vi "FPGAcode_check_velocity.vi"() -> ()   [LabVIEW 2015]
uses:
  <vilib>/Platform/TimedLoop/XDataNode/timing_clust.ctl
  <vilib>/Platform/TimedLoop/XDataNode/nitl_modes.ctl
  <vilib>/Platform/TimedLoop/XDataNode/wakeup.ctl
  <vilib>/rvi/eio/common/nirviEmuTemplateMethod_errors.vi
  <vilib>/rvi/Emulation/niFpgaGetClockAttributes.vi
  <vilib>/rvi/Emulation/niFpgaSctlEmulationGetInTimedLoop.vi
  <vilib>/rvi/Emulation/niFpgaEmulationReportErrorSimple.vi
  <vilib>/rvi/Emulation/niFpgaProcessEmulError.vi
  <vilib>/rvi/Emulation/niFpgaCriticalErrorInLSC.vi
  <vilib>/eio/EIONode/EIONode.xnode
  <vilib>/Platform/TimedLoop/XDataNode/XDataNode.xnode
  <vilib>/Platform/TimedLoop/XDataNode/XDNodeRunTimeDep.lvlib
panel:
  out "Check Data?":bool
  out "Filter":i16
  out "Vel Count 7":i32
  out "Vel Count 6":i32
  out "Vel Count 5":i32
  out "Vel Count 4":i32
  out "Vel Count 3":i32
  out "Vel Count 2":i32
  out "Vel Count 1":i32
  out "Filter 1 Detector 3 Correlation":i32
  in  "Filter 2 threshold":i32=1000
  out "Filter 2 Detector 3 Correlation":i32
  in  "Filter 1 threshold":i32=1000
  in  "Filter 3 threshold":i32=1000
  out "Filter 3 Detector 3 Correlation":i32
  in  "Filter 4 threshold":i32=1000
  out "Filter 4 Detector 3 Correlation":i32
  in  "Filter 5 threshold":i32
  out "Filter 5 Detector 3 Correlation":i32
  in  "Filter 6 threshold":i32
  out "Filter 6 Detector 3 Correlation":i32
  in  "Filter 7 threshold":i32
  out "Filter 7 Detector 3 Correlation":i32
  out "Plates":bool
  in  "High Charge Limit":i16
  in  "Low Charge Limit":i16
  in  "High Velocity Count":i32
  in  "Low Velocity Count":i32
  in  "High Mass Limit":i64
  in  "Low Mass Limit":i64
  in  "Mult1":fxp<+,16,7>
  out "Delay1":bool
  in  "One Shot":bool
  out "Not Armed?":bool
  in  "Reset One Shot":bool
  out "Del Not Armed?":bool
  out "IO Module\\AI 0":i16
  out "IO Module\\AI 1":i16
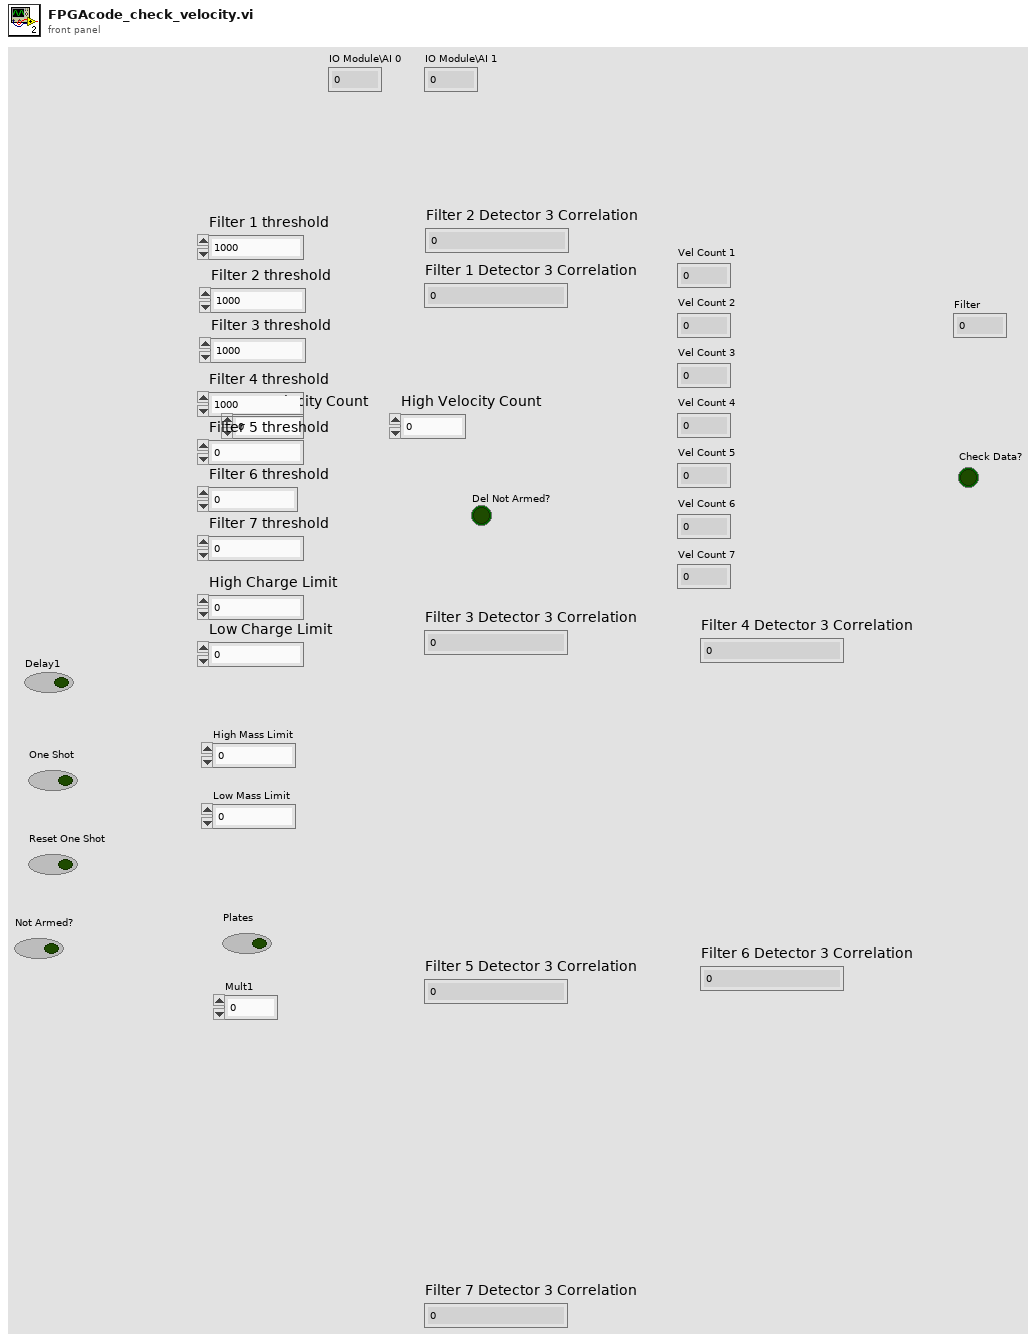
[diagram p1: front panel]
types:
  T1 = typedef "XDNodeRunTimeDep.lvlib/timing_clust.ctl" = cluster{"Expected End [f-1]":u64, "Actual End [f-1]":u64, "Finished Late? [f-1]":bool, "Expected End [i-1]":u64, "Actual End [i-1]":u64, "Finished Late? [i-1]":bool, "Expected Start [i]":u64, "Actual Start [i]":u64, "Expected Start [f]":u64, "Actual Start [f]":u64, "Source Name":string, "Structure Name":string, "Period":i64, "Deadline":i64, "Offset":i64, "Start":i64, "Priority":i32, "Timeout":i32, "Mode":T2, "Wakeup Reason":T3, "Error":errorcluster, "Source Type":string, "Secondary Source Type":string, "Global End Time":u64, "Global Start Time":u64, "Frame Duration":u64, "Iteration Duration":u64, "Assigned CPU":i32, "I/O Scan Engine Mode":u32}
  T2 = typedef "XDNodeRunTimeDep.lvlib/nitl_modes.ctl" = enum32{"No Change", "Process missed periods, maintain original phase", "Discard missed periods, maintain original phase", "Process missed periods, ignore original phase", "Discard missed periods, ignore original phase"}
  T3 = typedef "XDNodeRunTimeDep.lvlib/wakeup.ctl" = enum32{"Normal", "Aborted", "Asynchronous wakeup", "Timing source error", "Timed loop error", "Timeout"}
  T4 = cluster{"Separation cut off 1":i32, "Filter Number":i32, "Separation cut off 2":i32}
  T5 = cluster{"Old Average":i32, "New Average":i32, "Current State":u8, "Detector 1 Correlation":i32, "Detector 3 Correlation":i32, "Velocity Count":i32, "Detector Counter in":i32, "Timeout Count in":i32, "Measured Charge in":i32, "Filter Threshold":i32, "High Correlation in":i32, "Offset":i32, "Offset Average":i32, "Measured Velocity In":i32, "Mult Cluster":cluster{"Mult1":fxp<+,16,7>, "Mult1 Use?":bool}, "Final Delay Count In":u16, "Delay1 In":i32}
  T6 = cluster{"High Charge Limit":i16, "Low Charge Limit":i16, "Low Velocity Count":i32, "High Velocity Count":i32, "Low Velocity Count":i32, fxp<+,30,25>, "High Mass Limit":i64, "Low Mass Limit":i64}
  T7 = cluster{"Average Out":i32, "Next State":u8, "Velocity Count out":i32, "Detector counter out":i32, "Timeout count out":u32, "Measured Charge Out":i32, "High Correlation Out":i32, "Plates":bool, "Offset Out":i32, "Measured Velocity Out":i32, "Final Delay Count Out":u16, "Out1":bool, "Delay1":i32}
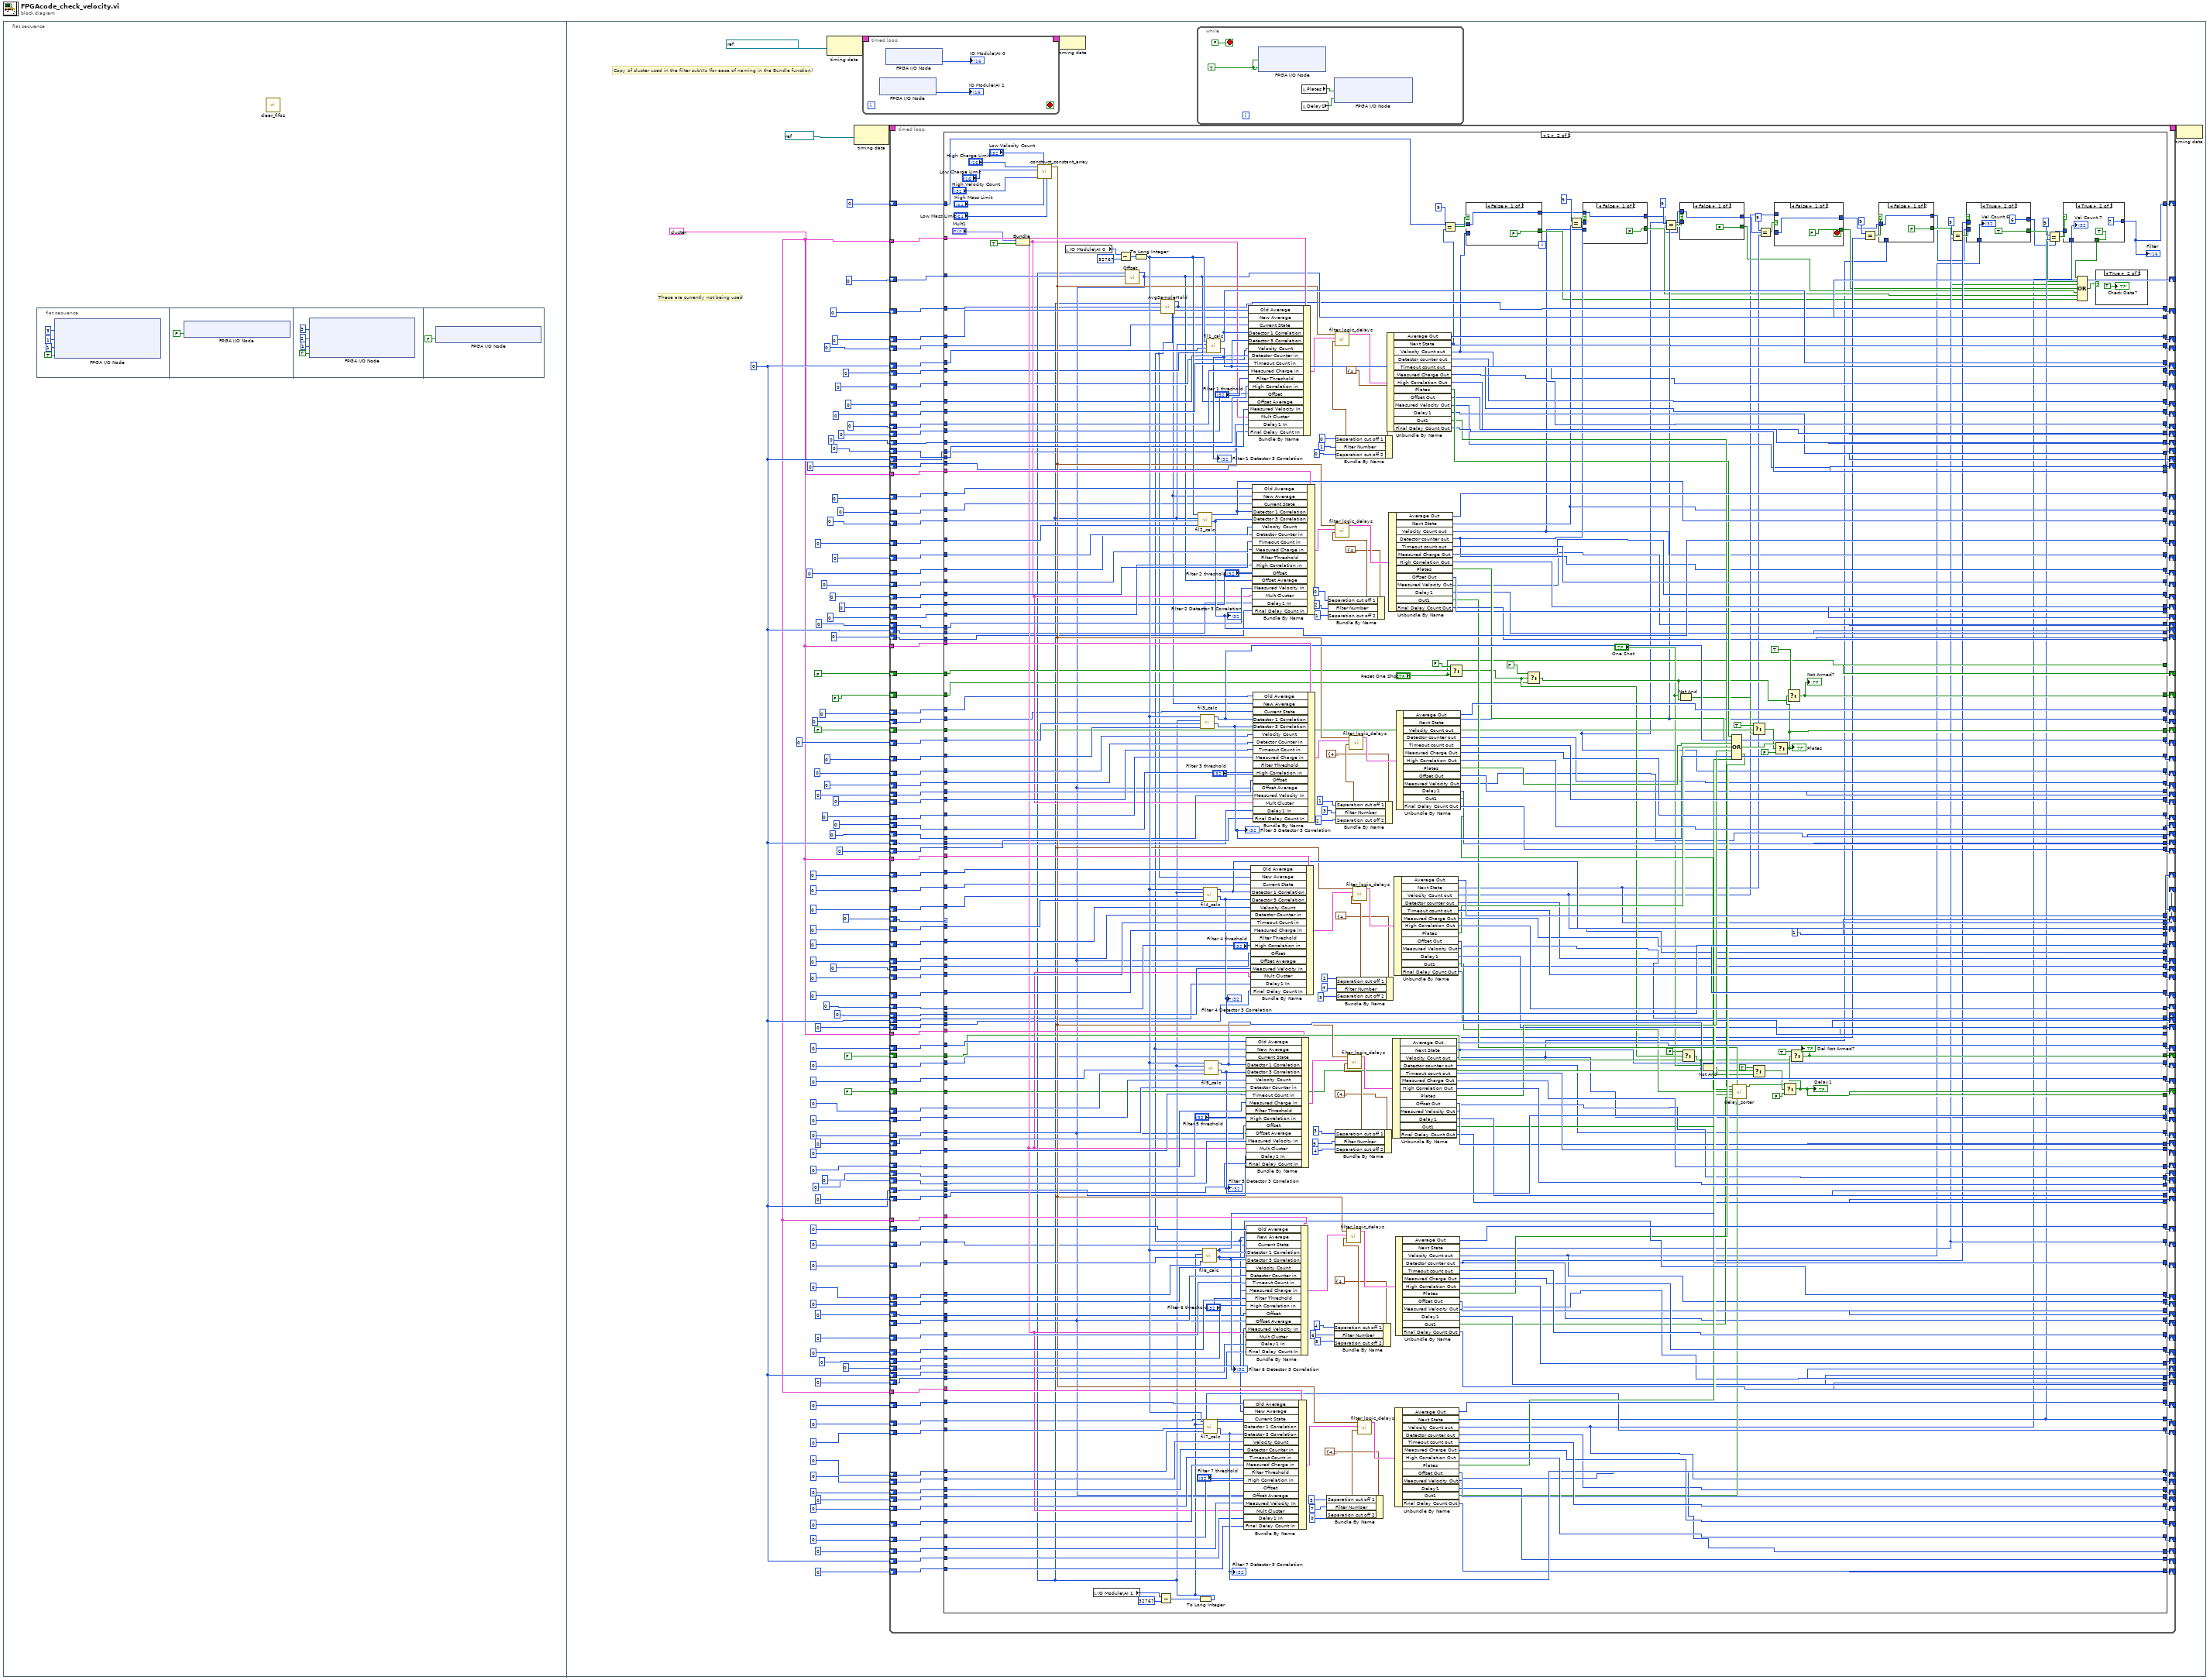
[diagram p0: block diagram]
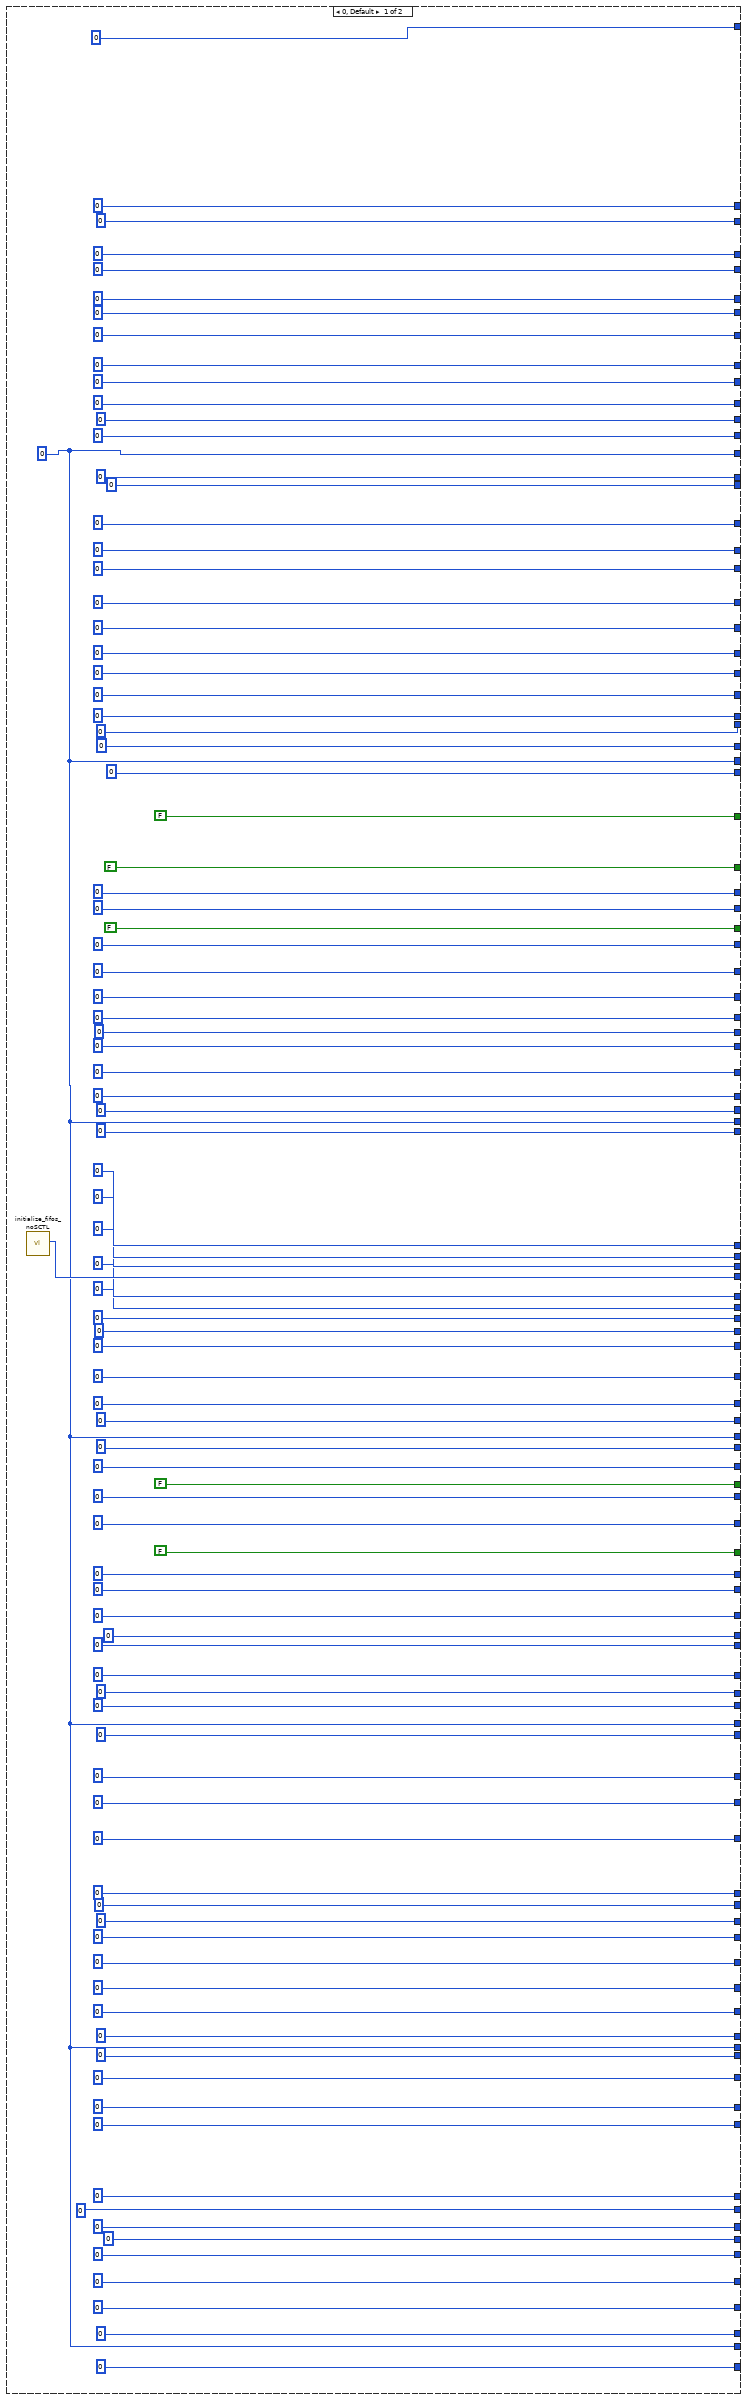
[diagram p2: hidden frame]
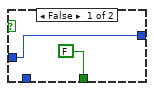
[diagram p4: hidden frame]
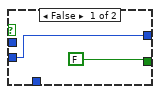
[diagram p5: hidden frame]
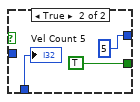
[diagram p6: hidden frame]
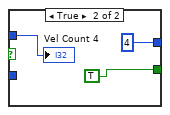
[diagram p7: hidden frame]
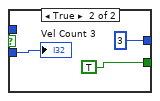
[diagram p8: hidden frame]
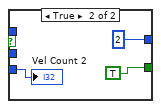
[diagram p9: hidden frame]
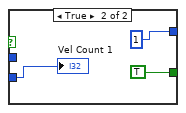
[diagram p10: hidden frame]
diagram:
  n1 = flat-sequence {
    frame #0 {
      n2 = flat-sequence {
        frame #0 {
          n3 = xnode "FPGA I/O Node"("IO Module\\User Command"=u8 3 ("IO Module\\User Command"), "IO Module\\User Data 0"=u8 1 ("IO Module\\User Data 0"), "IO Module\\User Data 1"=u8 1 ("IO Module\\User Data 1"), "IO Module\\User Command Commit"=TRUE ("IO Module\\User Command Commit")) -> ()  [unwired: 4 in, 4 out]
        }
        frame #1 {
          n4 = xnode "FPGA I/O Node"("IO Module\\User Command Commit"=FALSE ("IO Module\\User Command Commit")) -> ()  [unwired: 1 in, 1 out]
        }
        frame #2 {
          n5 = xnode "FPGA I/O Node"("IO Module\\User Command"=u8 3 ("IO Module\\User Command"), "IO Module\\User Data 0"=u8 2 ("IO Module\\User Data 0"), "IO Module\\User Data 1"=u8 1 ("IO Module\\User Data 1"), "IO Module\\User Command Commit"=TRUE ("IO Module\\User Command Commit")) -> ()  [unwired: 4 in, 4 out]
        }
        frame #3 {
          n6 = xnode "FPGA I/O Node"("IO Module\\User Command Commit"=FALSE ("IO Module\\User Command Commit")) -> ()  [unwired: 1 in, 1 out]
        }
      }
      n7 = call "clear_fifos.vi"() -> ()  [unwired: 1 in]
    }
    frame #1 {
      w16 = T5 {"Old Average"=0, "New Average"=0, "Current State"=0, "Detector 1 Correlation"=0, "Detector 3 Correlation"=0, "Velocity Count"=0, "Detector Counter in"=0, "Timeout Count in"=0, "Measured Charge in"=0, "Filter Threshold"=0, "High Correlation in"=0, "Offset"=0, "Offset Average"=0, "Measured Velocity In"=0, "Mult Cluster"={"Mult1"=0.0, "Mult1 Use?"=FALSE}, "Final Delay Count In"=0, "Delay1 In"=0} ("Variables Cluster")
      w19 = 0 ("Detector 1 Correlation Out")
      # "These are currently not being used"
      # "Copy of cluster used in the filter subVIs (for ease of naming in the Bundle function)"
      n8 = node-c288(refnum<k21> "IO Module\\Sample Clock" ("Source Name")) -> (w45:T1)
      n9 = node-c288(refnum<k21> "26MHz" ("Source Name")) -> (w109:T1)
      n10 = timed-loop {
        timing: w45 -> [_]
        timing-out: [_] -> w44
        stop <- _ stop-if-true
        n11 = xnode "FPGA I/O Node"() -> ("IO Module\\AI 2"=→"IO Module\\AI 1":u16)  [unwired: 1 in, 1 out]
        n12 = xnode "FPGA I/O Node"() -> ("IO Module\\AI 1"=→"IO Module\\AI 0":u16)  [unwired: 1 in, 1 out]
      }
      n13 = timed-loop {
        timing: w109 -> [_]
        timing-out: [_] -> w108
        shift-right: [w321] -> _
        shift-left: 0 ("Velocity Count out") -> [w243]
        shift-right: [w322] -> _
        shift-left: 0 ("Detector 1 Correlation out") -> [w244]
        shift-right: [w208] -> _
        shift-left: 0 ("Detector counter out") -> [w245]
        shift-right: [w239] -> _
        shift-left: 0 ("Next State") -> [w246]
        shift-right: [w207] -> _
        shift-left: 0 ("Detector 3 Correlation out") -> [w242]
        shift-right: [w320] -> _
        shift-left: 0 ("Timeout count out") -> [w241]
        shift-right: [w235] -> _
        shift-left: 0 ("Next State") -> [w238]
        shift-right: [w234] -> _
        shift-left: 0 ("Detector counter out") -> [w237]
        shift-right: [w206] -> _
        shift-left: 0 ("Detector 1 Correlation out") -> [w314]
        shift-right: [w311] -> _
        shift-left: 0 ("Velocity Count out") -> [w313]
        shift-right: [w310] -> _
        shift-left: u32 0 ("Detector 3 Correlation out") -> [w312]
        shift-right: [w305] -> _
        shift-left: 0 ("Timeout count out") -> [w306]
        shift-right: [w229] -> _
        shift-left: 0 ("Next State") -> [w232]
        shift-right: [w204] -> _
        shift-left: 0 ("Detector counter out") -> [w302]
        shift-right: [w300] -> _
        shift-left: 0 ("Detector 1 Correlation out") -> [w301]
        shift-right: [w298] -> _
        shift-left: u32 0 ("Velocity Count out") -> [w299]
        shift-right: [w203] -> _
        shift-left: 0 ("Detector 3 Correlation out") -> [w297]
        shift-right: [w296] -> _
        shift-left: 0 ("Timeout count out") -> [w231]
        shift-right: [w323] -> _
        shift-left: u8 0 ("High Correlation Out") -> [w326]
        shift-right: [w315] -> _
        shift-left: u8 0 ("High Correlation Out") -> [w316]
        shift-right: [w230] -> _
        shift-left: 0 ("High Correlation Out") -> [w233]
        shift-right: [w324] -> _
        shift-left: 0 ("Measured Charge Out") -> [w327]
        shift-right: [w317] -> _
        shift-left: 0 ("Measured Charge Out") -> [w318]
        shift-right: [w304] -> _
        shift-left: u8 0 ("Measured Charge Out") -> [w303]
        shift-right: [w194] -> _
        shift-left: 0 ("Output New Average") -> [w328]
        shift-right: [w240] -> _
        shift-left: w19 -> [w247]
        tunnel: w16 -> [w325]
        shift-right: [w205] -> _
        shift-left: 0 ("High Sample Out") -> [w308]
        shift-right: [w309] -> _
        shift-left: 0 ("High Correlation Out") -> [w236]
        tunnel: w16 -> [w319]
        tunnel: w16 -> [w307]
        shift-right: [w295] -> _
        shift-left: 0 ("Average Out") -> [w294]
        shift-right: [w293] -> _
        shift-left: u8 0 ("Next State") -> [w292]
        shift-right: [w225] -> _
        shift-left: 0 ("Detector 1 Correlation out") -> [w227]
        shift-right: [w224] -> _
        shift-left: 0 ("Detector 3 Correlation out") -> [w226]
        shift-right: [w202] -> _
        shift-left: 0 ("Velocity Count out") -> [w291]
        shift-right: [w290] -> _
        shift-left: 0 ("Detector counter out") -> [w289]
        shift-right: [w288] -> _
        shift-left: u32 0 ("Timeout count out") -> [w287]
        shift-right: [w201] -> _
        shift-left: 0 ("Measured Charge Out") -> [w286]
        shift-right: [w285] -> _
        shift-left: 0 ("High Correlation Out") -> [w228]
        tunnel: w16 -> [w284]
        shift-right: [w282] -> _
        shift-left: 0 ("Average Out") -> [w281]
        shift-right: [w280] -> _
        shift-left: u8 0 ("Next State") -> [w279]
        shift-right: [w220] -> _
        shift-left: 0 ("Detector 1 Correlation out") -> [w223]
        shift-right: [w219] -> _
        shift-left: 0 ("Detector 3 Correlation out") -> [w222]
        shift-right: [w200] -> _
        shift-left: 0 ("Velocity Count out") -> [w278]
        shift-right: [w277] -> _
        shift-left: 0 ("Detector counter out") -> [w276]
        shift-right: [w275] -> _
        shift-left: u32 0 ("Timeout count out") -> [w274]
        shift-right: [w199] -> _
        shift-left: 0 ("Measured Charge Out") -> [w273]
        shift-right: [w272] -> _
        shift-left: 0 ("High Correlation Out") -> [w221]
        tunnel: w16 -> [w283]
        shift-right: [w270] -> _
        shift-left: 0 ("Average Out") -> [w268]
        shift-right: [w269] -> _
        shift-left: u8 0 ("Next State") -> [w265]
        shift-right: [w215] -> _
        shift-left: 0 ("Detector 1 Correlation out") -> [w218]
        shift-right: [w214] -> _
        shift-left: 0 ("Detector 3 Correlation out") -> [w217]
        shift-right: [w197] -> _
        shift-left: 0 ("Velocity Count out") -> [w267]
        shift-right: [w264] -> _
        shift-left: _ -> [w266]
        shift-right: [w263] -> _
        shift-left: u32 0 ("Timeout count out") -> [w262]
        shift-right: [w198] -> _
        shift-left: 0 ("Measured Charge Out") -> [w261]
        shift-right: [w260] -> _
        shift-left: 0 ("High Correlation Out") -> [w216]
        tunnel: w16 -> [w271]
        shift-right: [w258] -> _
        shift-left: 0 ("Average Out") -> [w257]
        shift-right: [w256] -> _
        shift-left: u8 0 ("Next State") -> [w248]
        shift-right: [w210] -> _
        shift-left: 0 ("Detector 1 Correlation out") -> [w213]
        shift-right: [w209] -> _
        shift-left: 0 ("Detector 3 Correlation out") -> [w212]
        shift-right: [w196] -> _
        shift-left: 0 ("Velocity Count out") -> [w255]
        shift-right: [w254] -> _
        shift-left: 0 ("Detector counter out") -> [w253]
        shift-right: [w252] -> _
        shift-left: u32 0 ("Timeout count out") -> [w251]
        shift-right: [w195] -> _
        shift-left: 0 ("Measured Charge Out") -> [w250]
        shift-right: [w249] -> _
        shift-left: 0 ("High Correlation Out") -> [w211]
        tunnel: w16 -> [w259]
        shift-right: [w192] -> _
        shift-left: i16 0 -> [w193]
        shift-right: [w190] -> _
        shift-left: 0 -> [w191]
        shift-right: [w189] -> _
        shift-left: 0 -> [w186]
        shift-right: [w187] -> _
        shift-left: 0 -> [w188]
        shift-right: [w184] -> _
        shift-left: 0 ("Offset Out") -> [w185]
        shift-right: [w183] -> _
        shift-left: 0 ("Offset Out") -> [w182]
        shift-right: [w181] -> _
        shift-left: 0 ("Offset Out") -> [w180]
        shift-right: [w179] -> _
        shift-left: 0 ("Offset Out") -> [w178]
        shift-right: [w177] -> _
        shift-left: 0 ("Offset Out") -> [w176]
        shift-right: [w174] -> _
        shift-left: 0 -> [w175]
        shift-right: [w173] -> _
        shift-left: 0 -> [w162]
        shift-right: [w172] -> _
        shift-left: 0 -> [w163]
        shift-right: [w171] -> _
        shift-left: 0 -> [w164]
        shift-right: [w170] -> _
        shift-left: 0 -> [w165]
        shift-right: [w169] -> _
        shift-left: 0 -> [w166]
        shift-right: [w168] -> _
        shift-left: 0 ("Measured Velocity Out") -> [w167]
        shift-right: [w161] -> _
        shift-left: w19 -> [w159]
        shift-right: [w160] -> _
        shift-left: u32 0 ("Final Delay Count Out") -> [w158]
        shift-right: [w157] -> _
        shift-left: w19 -> [w155]
        shift-right: [w156] -> _
        shift-left: u32 0 ("Final Delay Count Out") -> [w154]
        shift-right: [w153] -> _
        shift-left: w19 -> [w151]
        shift-right: [w152] -> _
        shift-left: u32 0 ("Final Delay Count Out") -> [w150]
        shift-right: [w149] -> _
        shift-left: w19 -> [w147]
        shift-right: [w148] -> _
        shift-left: u32 0 ("Final Delay Count Out") -> [w146]
        shift-right: [w145] -> _
        shift-left: w19 -> [w143]
        shift-right: [w144] -> _
        shift-left: u32 0 ("Final Delay Count Out") -> [w142]
        shift-right: [w141] -> _
        shift-left: w19 -> [w139]
        shift-right: [w140] -> _
        shift-left: u32 0 ("Final Delay Count Out") -> [w138]
        shift-right: [w137] -> _
        shift-left: w19 -> [w135]
        shift-right: [w136] -> _
        shift-left: u32 0 ("Final Delay Count Out") -> [w134]
        shift-right: [w132] -> _
        shift-left: FALSE -> [w133]
        shift-right: [w131] -> _
        shift-left: FALSE ("f") -> [w130]
        shift-right: [w129] -> _
        shift-left: FALSE ("Reset One Shot") -> [w128]
        shift-right: [w124] -> _
        shift-left: FALSE -> [w127]
        shift-right: [w125] -> _
        shift-left: FALSE -> [w126]
        shift-right: [w123] -> _
        shift-left: i16 0 ("Filter") -> [w122]
        stop <- _ stop-if-true
        n14 = case shown="1" w193 {
          tunnel: w328 -> [_ w491]
          tunnel: w327 -> [_ w763]
          tunnel: w326 -> [_ w458]
          tunnel: w325 -> [_ w762]
          tunnel: [0 ("Average Out") w761] -> w324
          tunnel: [u16 0 ("Next State") w488] -> w323
          tunnel: [0 ("Detector counter out") w481] -> w322
          tunnel: [u32 0 ("Timeout count out") w760] -> w321
          tunnel: [0 ("High Correlation Out") w759] -> w320
          tunnel: w319 -> [_ w758]
          tunnel: w318 -> [_ w757]
          tunnel: [0 ("Average Out") w756] -> w317
          tunnel: w316 -> [_ w457]
          tunnel: [u16 0 ("Next State") w480] -> w315
          tunnel: w314 -> [_ w755]
          tunnel: w313 -> [_ w617]
          tunnel: w312 -> [_ w754]
          tunnel: [0 ("Detector counter out") w479] -> w311
          tunnel: [u32 0 ("Timeout count out") w753] -> w310
          tunnel: [0 ("High Correlation Out") w752] -> w309
          tunnel: w308 -> [_ w751]
          tunnel: w307 -> [_ w750]
          tunnel: w306 -> [_ w749]
          tunnel: [0 ("Average Out") w748] -> w305
          tunnel: [u16 0 ("Next State") w477] -> w304
          tunnel: w303 -> [_ w456]
          tunnel: w302 -> [_ w747]
          tunnel: w301 -> [_ w616]
          tunnel: [0 ("Detector counter out") w476] -> w300
          tunnel: w299 -> [_ w746]
          tunnel: [u32 0 ("Timeout count out") w745] -> w298
          tunnel: w297 -> [_ w744]
          tunnel: [0 ("High Correlation Out") w743] -> w296
          tunnel: [0 ("Average Out") w742] -> w295
          tunnel: w294 -> [_ w741]
          tunnel: [u16 0 ("Next State") w466] -> w293
          tunnel: w292 -> [_ w455]
          tunnel: w291 -> [_ w740]
          tunnel: [0 ("Detector counter out") w465] -> w290
          tunnel: w289 -> [_ w615]
          tunnel: [u32 0 ("Timeout count out") w739] -> w288
          tunnel: w287 -> [_ w738]
          tunnel: w286 -> [_ w737]
          tunnel: [0 ("High Correlation Out") w736] -> w285
          tunnel: w284 -> [_ w735]
          tunnel: w283 -> [_ w734]
          tunnel: [0 ("Average Out") w733] -> w282
          tunnel: w281 -> [_ w732]
          tunnel: [u16 0 ("Next State") w464] -> w280
          tunnel: w279 -> [_ w454]
          tunnel: w278 -> [_ w731]
          tunnel: [0 ("Detector counter out") w463] -> w277
          tunnel: w276 -> [_ w614]
          tunnel: [u32 0 ("Timeout count out") w730] -> w275
          tunnel: w274 -> [_ w729]
          tunnel: w273 -> [_ w728]
          tunnel: [0 ("High Correlation Out") w727] -> w272
          tunnel: w271 -> [_ w726]
          tunnel: [0 ("Average Out") w725] -> w270
          tunnel: [u16 0 ("Next State") w462] -> w269
          tunnel: w268 -> [_ w724]
          tunnel: w267 -> [_ w723]
          tunnel: w266 -> [_ w613]
          tunnel: w265 -> [_ w453]
          tunnel: [0 ("Detector counter out") w461] -> w264
          tunnel: [u32 0 ("Timeout count out") w722] -> w263
          tunnel: w262 -> [_ w721]
          tunnel: w261 -> [_ w720]
          tunnel: [0 ("High Correlation Out") w719] -> w260
          tunnel: w259 -> [_ w718]
          tunnel: [0 ("Average Out") w717] -> w258
          tunnel: w257 -> [_ w716]
          tunnel: [u16 0 ("Next State") w460] -> w256
          tunnel: w255 -> [_ w715]
          tunnel: [0 ("Detector counter out") w459] -> w254
          tunnel: w253 -> [_ w612]
          tunnel: [u32 0 ("Timeout count out") w714] -> w252
          tunnel: w251 -> [_ w713]
          tunnel: w250 -> [_ w712]
          tunnel: [0 ("High Correlation Out") w711] -> w249
          tunnel: w248 -> [_ w452]
          tunnel: w247 -> [_ w710]
          tunnel: w246 -> [_ w530]
          tunnel: w245 -> [_ w531]
          tunnel: w244 -> [_ w618]
          tunnel: w243 -> [_ w709]
          tunnel: w242 -> [_ w708]
          tunnel: w241 -> [_ w707]
          tunnel: [0 ("Detector 1 Correlation Out") w706] -> w240
          tunnel: [0 ("Detector 3 Correlation Out") w705] -> w239
          tunnel: w238 -> [_ w704]
          tunnel: w237 -> [_ w703]
          tunnel: w236 -> [_ w702]
          tunnel: [0 ("Detector 1 Correlation Out") w701] -> w235
          tunnel: [0 ("Detector 3 Correlation Out") w700] -> w234
          tunnel: w233 -> [_ w699]
          tunnel: w232 -> [_ w698]
          tunnel: w231 -> [_ w697]
          tunnel: [0 ("Detector 1 Correlation Out") w696] -> w230
          tunnel: [0 ("Detector 3 Correlation Out") w695] -> w229
          tunnel: w228 -> [_ w694]
          tunnel: w227 -> [_ w693]
          tunnel: w226 -> [_ w692]
          tunnel: [0 ("Detector 1 Correlation Out") w691] -> w225
          tunnel: [0 ("Detector 3 Correlation Out") w690] -> w224
          tunnel: w223 -> [_ w689]
          tunnel: w222 -> [_ w688]
          tunnel: w221 -> [_ w687]
          tunnel: [0 ("Detector 1 Correlation Out") w686] -> w220
          tunnel: [0 ("Detector 3 Correlation Out") w685] -> w219
          tunnel: w218 -> [_ w684]
          tunnel: w217 -> [_ w683]
          tunnel: w216 -> [_ w682]
          tunnel: [0 ("Detector 1 Correlation Out") w681] -> w215
          tunnel: [0 ("Detector 3 Correlation Out") w680] -> w214
          tunnel: w213 -> [_ w679]
          tunnel: w212 -> [_ w678]
          tunnel: w211 -> [_ w677]
          tunnel: [0 ("Detector 1 Correlation Out") w565] -> w210
          tunnel: [0 ("Detector 3 Correlation Out") w676] -> w209
          tunnel: [0 ("Velocity Count out") w444] -> w208
          tunnel: [0 ("Measured Charge Out") w675] -> w207
          tunnel: [0 ("Velocity Count out") w441] -> w206
          tunnel: [0 ("Measured Charge Out") w674] -> w205
          tunnel: [0 ("Velocity Count out") w440] -> w204
          tunnel: [0 ("Measured Charge Out") w673] -> w203
          tunnel: [0 ("Velocity Count out") w438] -> w202
          tunnel: [0 ("Measured Charge Out") w672] -> w201
          tunnel: [0 ("Velocity Count out") w436] -> w200
          tunnel: [0 ("Measured Charge Out") w671] -> w199
          tunnel: [0 ("Measured Charge Out") w670] -> w198
          tunnel: [0 ("Velocity Count out") w435] -> w197
          tunnel: [0 ("Velocity Count out") w432] -> w196
          tunnel: [0 ("Measured Charge Out") w669] -> w195
          tunnel: [0 ("Output New Average") w490] -> w194
          tunnel: [w422 i16 1 ("Output State")] -> w192
          tunnel: w191 -> [_ w611]
          tunnel: [0 ("Offset Out") w610] -> w190
          tunnel: [0 ("Offset Out") w609] -> w189
          tunnel: w188 -> [_ w494]
          tunnel: [0 ("Output New Average") w493] -> w187
          tunnel: w186 -> [_ w608]
          tunnel: w185 -> [_ w607]
          tunnel: [0 ("Offset Out") w606] -> w184
          tunnel: [0 ("Offset Out") w605] -> w183
          tunnel: w182 -> [_ w604]
          tunnel: [0 ("Offset Out") w603] -> w181
          tunnel: w180 -> [_ w602]
          tunnel: [0 ("Offset Out") w601] -> w179
          tunnel: w178 -> [_ w600]
          tunnel: [0 ("Offset Out") w599] -> w177
          tunnel: w176 -> [_ w598]
          tunnel: w175 -> [_ w593]
          tunnel: [0 ("Measured Velocity Out") w489] -> w174
          tunnel: [0 ("Measured Velocity Out") w478] -> w173
          tunnel: [0 ("Measured Velocity Out") w475] -> w172
          tunnel: [0 ("Measured Velocity Out") w586] -> w171
          tunnel: [0 ("Measured Velocity Out") w585] -> w170
          tunnel: [0 ("Measured Velocity Out") w584] -> w169
          tunnel: [0 ("Measured Velocity Out") w583] -> w168
          tunnel: w167 -> [_ w592]
          tunnel: w166 -> [_ w591]
          tunnel: w165 -> [_ w590]
          tunnel: w164 -> [_ w589]
          tunnel: w163 -> [_ w588]
          tunnel: w162 -> [_ w587]
          tunnel: [w335 w560] -> w161
          tunnel: [u32 0 ("Final Delay Count Out") w578] -> w160
          tunnel: w159 -> [_ w577]
          tunnel: w158 -> [_ w576]
          tunnel: [w335 w575] -> w157
          tunnel: [u32 0 ("Final Delay Count Out") w574] -> w156
          tunnel: w155 -> [_ w573]
          tunnel: w154 -> [_ w572]
          tunnel: [w335 w559] -> w153
          tunnel: [u32 0 ("Final Delay Count Out") w571] -> w152
          tunnel: w151 -> [_ w552]
          tunnel: w150 -> [_ w570]
          tunnel: [w335 w558] -> w149
          tunnel: [u32 0 ("Final Delay Count Out") w569] -> w148
          tunnel: w147 -> [_ w551]
          tunnel: w146 -> [_ w568]
          tunnel: [w335 w557] -> w145
          tunnel: [u32 0 ("Final Delay Count Out") w567] -> w144
          tunnel: w143 -> [_ w550]
          tunnel: w142 -> [_ w566]
          tunnel: [w335 w556] -> w141
          tunnel: [u32 0 ("Final Delay Count Out") w564] -> w140
          tunnel: w139 -> [_ w549]
          tunnel: w138 -> [_ w563]
          tunnel: [w335 w555] -> w137
          tunnel: [u32 0 ("Final Delay Count Out") w562] -> w136
          tunnel: w135 -> [_ w548]
          tunnel: w134 -> [_ w561]
          tunnel: w133 -> [_ w496]
          tunnel: [FALSE ("t") w516] -> w132
          tunnel: [FALSE ("f") w528] -> w131
          tunnel: w130 -> [_ w527]
          tunnel: [FALSE ("Reset One Shot") "Reset One Shot"] -> w129
          tunnel: w128 -> [_ w514]
          tunnel: w127 -> [_ w497]
          tunnel: w126 -> [_ w503]
          tunnel: [FALSE ("Delay1") w502] -> w125
          tunnel: [FALSE w499] -> w124
          tunnel: [i16 0 ("Filter") w430] -> w123
          tunnel: w122 -> [_ w442]
          frame 0, Default {
            w335 = 0
            n15 = call "initialize_fifos_noSCTL.vi"() -> ("Output State"=w422:i16)  [unwired: 11 in]
          }
          frame 1 {
            n16 = Bundle("Mult1"="Mult1", TRUE) -> (w579:cluster{"Mult1":fxp<+,16,7>, bool})  [unwired: 1 in]
            n17 = call "construct_constant_array.vi"("Low Mass Limit"="Low Mass Limit", "High Mass Limit"="High Mass Limit", "Low Velocity Count"="Low Velocity Count", "High Velocity Count"="High Velocity Count", "Low Charge Limit"="Low Charge Limit", "High Charge Limit"="High Charge Limit") -> ("constants cluster"=w580:T6)  [unwired: 5 in]
            n18 = local read "IO Module\\AI 0"() -> (w427:i16)
            n19 = local read "IO Module\\AI 1"() -> (w424:i16)
            n20 = Subtract(x=w427, y=i16 32767) -> (x-y=w428:i16)
            n21 = To Long Integer(number=w428) -> (32bit integer=w627:i32)
            n22 = Subtract(x=w424, y=i16 32767) -> (x-y=w423:i16)
            n23 = To Long Integer(number=w423) -> (32bit integer=w492:i32)
            n24 = call "Offset.vi"("Previous Average"=w494, "Input Value"=w492) -> ("Output New Average"=w493:i32)  [unwired: 9 in]
            n25 = call "AvgSampleHold.vi"("Previous Average"=w491, "Input Value"=w492) -> ("Output New Average"=w490:i32)  [unwired: 9 in]
            n26 = call "fil2_calc.vi"("Detector 3 Correlation In"=w703, "Detector 1 Correlation In"=w704, "AI1"=w492, "AI0"=w627) -> ("Detector 3 Correlation Out"=w700:i32, "Detector 1 Correlation Out"=w701:i32)  [unwired: 4 in]
            "Filter 2 Detector 3 Correlation" <- w700
            n27 = call "fil3_calc.vi"("Detector 3 Correlation In"=w698, "Detector 1 Correlation In"=w699, "AI1"=w492, "AI0"=w627) -> ("Detector 3 Correlation Out"=w695:i32, "Detector 1 Correlation Out"=w696:i32)  [unwired: 4 in]
            "Filter 3 Detector 3 Correlation" <- w695
            n28 = call "fil6_calc.vi"("Detector 3 Correlation In"=w683, "Detector 1 Correlation In"=w684, "AI1"=w492, "AI0"=w627) -> ("Detector 3 Correlation Out"=w680:i32, "Detector 1 Correlation Out"=w681:i32)  [unwired: 4 in]
            "Filter 6 Detector 3 Correlation" <- w680
            n29 = call "fil4_calc.vi"("Detector 3 Correlation In"=w692, "Detector 1 Correlation In"=w693, "AI1"=w492, "AI0"=w627) -> ("Detector 3 Correlation Out"=w690:i32, "Detector 1 Correlation Out"=w691:i32)  [unwired: 4 in]
            "Filter 4 Detector 3 Correlation" <- w690
            n30 = call "fil7_calc.vi"("Detector 3 Correlation In"=w678, "Detector 1 Correlation In"=w679, "AI1"=w492, "AI0"=w627) -> ("Detector 3 Correlation Out"=w676:i32, "Detector 1 Correlation Out"=w565:i32)  [unwired: 4 in]
            "Filter 7 Detector 3 Correlation" <- w676
            n31 = call "fil5_calc.vi"("Detector 3 Correlation In"=w688, "Detector 1 Correlation In"=w689, "AI1"=w492, "AI0"=w627) -> ("Detector 3 Correlation Out"=w685:i32, "Detector 1 Correlation Out"=w686:i32)  [unwired: 4 in]
            "Filter 5 Detector 3 Correlation" <- w685
            n32 = call "fil1_calc.vi"("Detector 3 Correlation In"=w530, "Detector 1 Correlation In"=w710, "AI1"=w492, "AI0"=w627) -> ("Detector 3 Correlation Out"=w705:i32, "Detector 1 Correlation Out"=w706:i32)  [unwired: 4 in]
            "Filter 1 Detector 3 Correlation" <- w705
            n33 = Bundle By Name(cluster=w718, "Old Average"=w716, "New Average"=w490, "Current State"=w452, "Detector 1 Correlation"=w565, "Detector 3 Correlation"=w676, "Velocity Count"=w715, "Detector Counter in"=w612, "Timeout Count in"=w713, "Measured Charge in"=w712, "Filter Threshold"="Filter 7 threshold", "High Correlation in"=w677, "Offset"=w598, "Offset Average"=w493, "Measured Velocity In"=w592, "Mult Cluster"=w579, "Delay1 In"=w548, "Final Delay Count In"=w561) -> (w518:T5)
            n34 = Bundle By Name(cluster=w726, "Old Average"=w724, "New Average"=w490, "Current State"=w453, "Detector 1 Correlation"=w681, "Detector 3 Correlation"=w680, "Velocity Count"=w723, "Detector Counter in"=w613, "Timeout Count in"=w721, "Measured Charge in"=w720, "Filter Threshold"="Filter 6 threshold", "High Correlation in"=w682, "Offset"=w600, "Offset Average"=w493, "Measured Velocity In"=w591, "Mult Cluster"=w579, "Delay1 In"=w549, "Final Delay Count In"=w563) -> (w519:T5)
            n35 = Bundle By Name(cluster=w734, "Old Average"=w732, "New Average"=w490, "Current State"=w454, "Detector 1 Correlation"=w686, "Detector 3 Correlation"=w685, "Velocity Count"=w731, "Detector Counter in"=w614, "Timeout Count in"=w729, "Measured Charge in"=w728, "Filter Threshold"="Filter 5 threshold", "High Correlation in"=w687, "Offset"=w602, "Offset Average"=w493, "Measured Velocity In"=w590, "Mult Cluster"=w579, "Delay1 In"=w550, "Final Delay Count In"=w566) -> (w520:T5)
            n36 = Bundle By Name(cluster=w762, "Old Average"=w763, "New Average"=w490, "Current State"=w458, "Detector 1 Correlation"=w706, "Detector 3 Correlation"=w705, "Velocity Count"=w531, "Detector Counter in"=w618, "Timeout Count in"=w709, "Measured Charge in"=w708, "Filter Threshold"="Filter 1 threshold", "High Correlation in"=w707, "Offset"=w611, "Offset Average"=w493, "Measured Velocity In"=w593, "Mult Cluster"=w579, "Delay1 In"=w577, "Final Delay Count In"=w576) -> (w524:T5)
            n37 = Bundle By Name(cluster=w735, "Old Average"=w741, "New Average"=w490, "Current State"=w455, "Detector 1 Correlation"=w691, "Detector 3 Correlation"=w690, "Velocity Count"=w740, "Detector Counter in"=w615, "Timeout Count in"=w738, "Measured Charge in"=w737, "Filter Threshold"="Filter 4 threshold", "High Correlation in"=w694, "Offset"=w604, "Offset Average"=w493, "Measured Velocity In"=w589, "Mult Cluster"=w579, "Delay1 In"=w551, "Final Delay Count In"=w568) -> (w521:T5)
            n38 = Bundle By Name(cluster=w758, "Old Average"=w757, "New Average"=w490, "Current State"=w457, "Detector 1 Correlation"=w701, "Detector 3 Correlation"=w700, "Velocity Count"=w755, "Detector Counter in"=w617, "Timeout Count in"=w754, "Measured Charge in"=w751, "Filter Threshold"="Filter 2 threshold", "High Correlation in"=w702, "Offset"=w608, "Offset Average"=w493, "Measured Velocity In"=w587, "Mult Cluster"=w579, "Delay1 In"=w573, "Final Delay Count In"=w572) -> (w523:T5)
            n39 = Bundle By Name(cluster=w750, "Old Average"=w749, "New Average"=w490, "Current State"=w456, "Detector 1 Correlation"=w696, "Detector 3 Correlation"=w695, "Velocity Count"=w747, "Detector Counter in"=w616, "Timeout Count in"=w746, "Measured Charge in"=w744, "Filter Threshold"="Filter 3 threshold", "High Correlation in"=w697, "Offset"=w607, "Offset Average"=w493, "Measured Velocity In"=w588, "Mult Cluster"=w579, "Delay1 In"=w552, "Final Delay Count In"=w570) -> (w522:T5)
            n40 = Bundle By Name(cluster=T4 {"Separation cut off 1"=4, "Filter Number"=5, "Separation cut off 2"=6} ("Filter Specific Constants"), "Separation cut off 1"=5, "Filter Number"=7, "Separation cut off 2"=0) -> (w534:T4)
            n41 = Bundle By Name(cluster=T4 {"Separation cut off 1"=4, "Filter Number"=5, "Separation cut off 2"=6} ("Filter Specific Constants"), "Separation cut off 1"=0, "Filter Number"=2, "Separation cut off 2"=1) -> (w660:T4)
            n42 = Bundle By Name(cluster=T4 {"Separation cut off 1"=4, "Filter Number"=5, "Separation cut off 2"=6} ("Filter Specific Constants"), "Separation cut off 1"=4, "Filter Number"=6, "Separation cut off 2"=5) -> (w650:T4)
            n43 = call "filter_logic_delays.vi"("Filter Specific Constants"=w660, "Variables Cluster"=w523, "controls cluster"=w580) -> ("Output Cluster"=w667:T7)  [unwired: 8 in]
            n44 = Bundle By Name(cluster=T4 {"Separation cut off 1"=4, "Filter Number"=5, "Separation cut off 2"=6} ("Filter Specific Constants"), "Separation cut off 1"=3, "Filter Number"=5, "Separation cut off 2"=4) -> (w652:T4)
            n45 = Bundle By Name(cluster=T4 {"Separation cut off 1"=4, "Filter Number"=5, "Separation cut off 2"=6} ("Filter Specific Constants"), "Separation cut off 1"=0, "Filter Number"=1, "Separation cut off 2"=0) -> (w658:T4)
            n46 = call "filter_logic_delays.vi"("Filter Specific Constants"=w658, "Variables Cluster"=w524, "controls cluster"=w580) -> ("Output Cluster"=w657:T7)  [unwired: 8 in]
            n47 = Bundle By Name(cluster=T4 {"Separation cut off 1"=4, "Filter Number"=5, "Separation cut off 2"=6} ("Filter Specific Constants"), "Separation cut off 1"=1, "Filter Number"=3, "Separation cut off 2"=2) -> (w656:T4)
            n48 = Bundle By Name(cluster=T4 {"Separation cut off 1"=4, "Filter Number"=5, "Separation cut off 2"=6} ("Filter Specific Constants"), "Separation cut off 1"=2, "Filter Number"=4, "Separation cut off 2"=3) -> (w654:T4)
            n49 = call "filter_logic_delays.vi"("Filter Specific Constants"=w650, "Variables Cluster"=w519, "controls cluster"=w580) -> ("Output Cluster"=w649:T7)  [unwired: 8 in]
            n50 = call "filter_logic_delays.vi"("Filter Specific Constants"=w652, "Variables Cluster"=w520, "controls cluster"=w580) -> ("Output Cluster"=w651:T7)  [unwired: 8 in]
            n51 = call "filter_logic_delays.vi"("Filter Specific Constants"=w656, "Variables Cluster"=w522, "controls cluster"=w580) -> ("Output Cluster"=w655:T7)  [unwired: 8 in]
            n52 = call "filter_logic_delays.vi"("Filter Specific Constants"=w654, "Variables Cluster"=w521, "controls cluster"=w580) -> ("Output Cluster"=w653:T7)  [unwired: 8 in]
            n53 = call "filter_logic_delays.vi"("Filter Specific Constants"=w534, "Variables Cluster"=w518, "controls cluster"=w580) -> ("Output Cluster"=w659:T7)  [unwired: 8 in]
            n54 = Unbundle By Name(w657) -> ("Average Out"=w761:i32, "Next State"=w488:u8, "Velocity Count out"=w444:i32, "Detector counter out"=w481:i32, "Timeout count out"=w760:u32, "Measured Charge Out"=w675:i32, "High Correlation Out"=w759:i32, "Plates"=w625:bool, "Offset Out"=w610:i32, "Measured Velocity Out"=w489:i32, "Delay1"=w560:i32, "Out1"=w554:bool, "Final Delay Count Out"=w578:u16)
            n55 = Unbundle By Name(w667) -> ("Average Out"=w756:i32, "Next State"=w480:u8, "Velocity Count out"=w441:i32, "Detector counter out"=w479:i32, "Timeout count out"=w753:u32, "Measured Charge Out"=w674:i32, "High Correlation Out"=w752:i32, "Plates"=w624:bool, "Offset Out"=w609:i32, "Measured Velocity Out"=w478:i32, "Delay1"=w575:i32, "Out1"=w553:bool, "Final Delay Count Out"=w574:u16)
            n56 = Unbundle By Name(w651) -> ("Average Out"=w733:i32, "Next State"=w464:u8, "Velocity Count out"=w436:i32, "Detector counter out"=w463:i32, "Timeout count out"=w730:u32, "Measured Charge Out"=w671:i32, "High Correlation Out"=w727:i32, "Plates"=w621:bool, "Offset Out"=w603:i32, "Measured Velocity Out"=w585:i32, "Delay1"=w557:i32, "Out1"=w544:bool, "Final Delay Count Out"=w567:u16)
            n57 = Unbundle By Name(w653) -> ("Average Out"=w742:i32, "Next State"=w466:u8, "Velocity Count out"=w438:i32, "Detector counter out"=w465:i32, "Timeout count out"=w739:u32, "Measured Charge Out"=w672:i32, "High Correlation Out"=w736:i32, "Plates"=w622:bool, "Offset Out"=w605:i32, "Measured Velocity Out"=w586:i32, "Delay1"=w558:i32, "Out1"=w545:bool, "Final Delay Count Out"=w569:u16)
            n58 = Unbundle By Name(w659) -> ("Average Out"=w717:i32, "Next State"=w460:u8, "Velocity Count out"=w432:i32, "Detector counter out"=w459:i32, "Timeout count out"=w714:u32, "Measured Charge Out"=w669:i32, "High Correlation Out"=w711:i32, "Plates"=w619:bool, "Offset Out"=w599:i32, "Measured Velocity Out"=w583:i32, "Delay1"=w555:i32, "Out1"=w543:bool, "Final Delay Count Out"=w562:u16)
            n59 = Unbundle By Name(w649) -> ("Average Out"=w725:i32, "Next State"=w462:u8, "Velocity Count out"=w435:i32, "Detector counter out"=w461:i32, "Timeout count out"=w722:u32, "Measured Charge Out"=w670:i32, "High Correlation Out"=w719:i32, "Plates"=w620:bool, "Offset Out"=w601:i32, "Measured Velocity Out"=w584:i32, "Delay1"=w556:i32, "Out1"=w542:bool, "Final Delay Count Out"=w564:u16)
            n60 = Unbundle By Name(w655) -> ("Average Out"=w748:i32, "Next State"=w477:u8, "Velocity Count out"=w440:i32, "Detector counter out"=w476:i32, "Timeout count out"=w745:u32, "Measured Charge Out"=w673:i32, "High Correlation Out"=w743:i32, "Plates"=w623:bool, "Offset Out"=w606:i32, "Measured Velocity Out"=w475:i32, "Delay1"=w559:i32, "Out1"=w546:bool, "Final Delay Count Out"=w571:u16)
            n61 = Equal?(x=u8 9, y=w488) -> (x = y?=w486:bool)
            n62 = Select(t=FALSE, s=w514, f="Reset One Shot") -> (s? t:f=w505:bool)
            n63 = case shown="False" w486 {
              tunnel: [FALSE TRUE] -> w445
              tunnel: w444 -> [_ w798]
              tunnel: [w795 i16 1 ("Filter")] -> w443
              tunnel: w442 -> [w795 _]
              frame False {
              }
              frame True {
                "Vel Count 1" <- w798
              }
            }
            n64 = Select(t=FALSE, s=w505, f=w496) -> (s? t:f=w517:bool)
            n65 = Equal?(x=u8 9, y=w480) -> (x = y?=w484:bool)
            n66 = case shown="False" w484 {
              tunnel: w479 -> [_ _]
              tunnel: [FALSE TRUE] -> w446
              tunnel: w443 -> [w790 _]
              tunnel: w441 -> [_ w793]
              tunnel: [w790 i16 2 ("Filter")] -> w439
              frame False {
              }
              frame True {
                "Vel Count 2" <- w793
              }
            }
            n67 = Equal?(x=u8 9, y=w477) -> (x = y?=w483:bool)
            n68 = Not And(1:w517, 2:"One Shot") -> (0:w508:bool)
            n69 = case shown="False" w483 {
              tunnel: [FALSE TRUE] -> w447
              tunnel: w440 -> [_ w788]
              tunnel: [w785 i16 3 ("Filter")] -> w437
              tunnel: w439 -> [w785 _]
              frame False {
              }
              frame True {
                "Vel Count 3" <- w788
              }
            }
            n70 = Select(t=FALSE, s=w505, f=w497) -> (s? t:f=w500:bool)
            n71 = Not And(1:w500, 2:"One Shot") -> (0:w506:bool)
            n72 = Compound Arithmetic op=OR(w625, w624, w623, w622, w621, w620, w619) -> (w533:bool)
            n73 = call "delay_sorter.vi"("Out1 1"=w554, "Out1 2"=w553, "Out1 3"=w546, "Out1 4"=w545, "Out1 5"=w544, "Out1 6"=w542, "Out1 7"=w543) -> ("Delay1"=w510:bool)  [unwired: 8 in]
            n74 = Select(t=TRUE, s=w527, f=w508) -> (s? t:f=w525:bool)
            n75 = Select(t=TRUE, s=w503, f=w506) -> (s? t:f=w512:bool)
            n76 = Equal?(x=u8 9, y=w466) -> (x = y?=w473:bool)
            n77 = case shown="False" w473 {
              tunnel: [FALSE TRUE] -> w448
              tunnel: [w780 i16 4 ("Filter")] -> w433
              tunnel: w438 -> [_ w782]
              tunnel: w437 -> [w780 _]
              frame False {
              }
              frame True {
                "Vel Count 4" <- w782
              }
            }
            n78 = Select(t=w533, s=w525, f=FALSE) -> (s? t:f=w528:bool)
            "Plates" <- w528
            n79 = Select(t=w510, s=w512, f=FALSE) -> (s? t:f=w502:bool)
            "Delay1" <- w502
            n80 = Select(t=TRUE, s=w528, f=w517) -> (s? t:f=w516:bool)
            "Not Armed?" <- w516
            n81 = Select(t=TRUE, s=w502, f=w500) -> (s? t:f=w499:bool)
            "Del Not Armed?" <- w499
            n82 = Equal?(x=u8 9, y=w464) -> (x = y?=w472:bool)
            n83 = case shown="False" w472 {
              tunnel: [FALSE TRUE] -> w449
              tunnel: w436 -> [_ w778]
              tunnel: [w775 i16 5 ("Filter")] -> w434
              tunnel: w433 -> [w775 _]
              frame False {
              }
              frame True {
                "Vel Count 5" <- w778
              }
            }
            n84 = Equal?(x=u8 9, y=w462) -> (x = y?=w469:bool)
            n85 = case shown="True" w469 {
              tunnel: w461 -> [_ _]
              tunnel: [FALSE TRUE] -> w450
              tunnel: w435 -> [_ w773]
              tunnel: [w770 i16 6 ("Filter")] -> w431
              tunnel: w434 -> [w770 _]
              frame False {
              }
              frame True {
                "Vel Count 6" <- w773
              }
            }
            n86 = Equal?(x=u8 9, y=w460) -> (x = y?=w468:bool)
            n87 = case shown="True" w468 {
              tunnel: [FALSE TRUE] -> w451
              tunnel: [w765 i16 7 ("Filter")] -> w430
              tunnel: w432 -> [_ w767]
              tunnel: w431 -> [w765 _]
              frame False {
              }
              frame True {
                "Vel Count 7" <- w767
              }
            }
            "Filter" <- w430
            n88 = Compound Arithmetic op=OR(w451, w450, w449, w448, w447, w446, w445) -> (w429:bool)
            n89 = case shown="True" w429 {
              frame False {
              }
              frame True {
                "Check Data?" <- TRUE ("Check Data?")
              }
            }
          }
        }
      }
      n90 = node-c288(w44) -> ()
      n91 = while {
        stop <- FALSE stop-if-true
        w120 = TRUE ("IO Module\\PFI Enable")
        n92 = xnode "FPGA I/O Node"("IO Module\\PFI 0 WE"=w120, "IO Module\\PFI 1 WE"=w120) -> ()  [unwired: 2 in, 2 out]
        n93 = local read "Plates"() -> (w119:bool)
        n94 = local read "Delay1"() -> (w118:bool)
        n95 = xnode "FPGA I/O Node"("IO Module\\PFI 0 Wr Data"=w119, "IO Module\\PFI 1 Wr Data"=w118) -> ()  [unwired: 2 in, 2 out]
      }
      n96 = node-c288(w108) -> ()
    }
  }
